vi "DataScope.vi"() -> ()   [LabVIEW 2020]
panel:
  in  "REF 종료점":u16=620
  in  "REF 시작점":u16=320
  in  "노이즈 수량":u16=255
  out "스톡스 인덱스":u32
  out "안티스톡스 인덱스":i32
  out "XY Graph":cluster{"Y":dbl[], "Y":dbl[]}[](graph) caption="XY 그래프"
  in  "거리해상도":string(combo)="5" caption="거리 해상도"
  in  "측정 거리":string(combo)="4" caption="측정 최대 거리"
  out "S문자열":string caption="스톡스 파일"
  out "AS문자열":string caption="안티스톡스 파일"
  in  "종료":bool
  in  "다음 데이터":bool
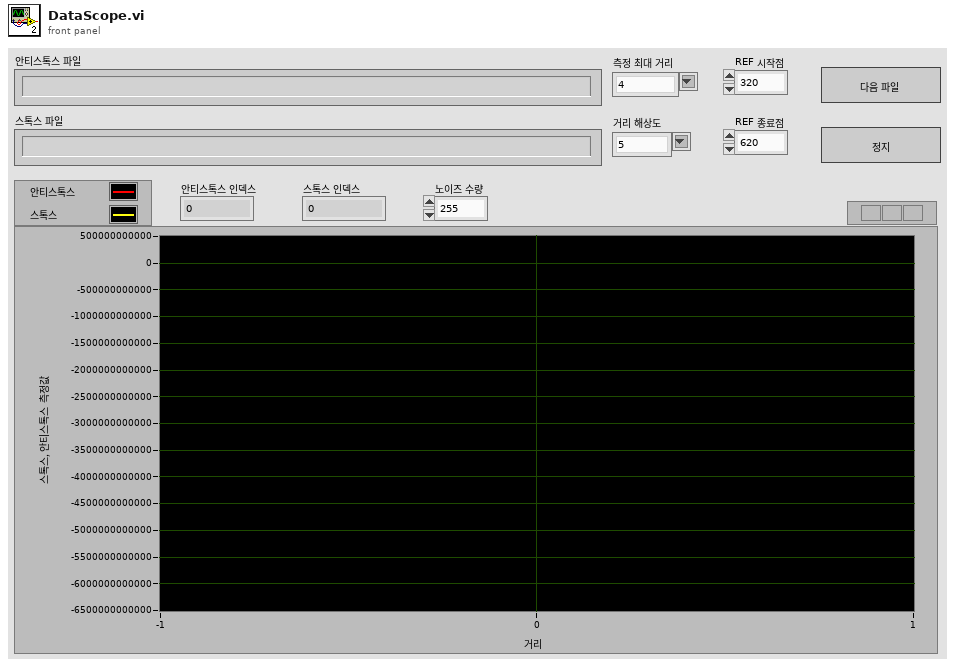
[diagram p1: front panel]
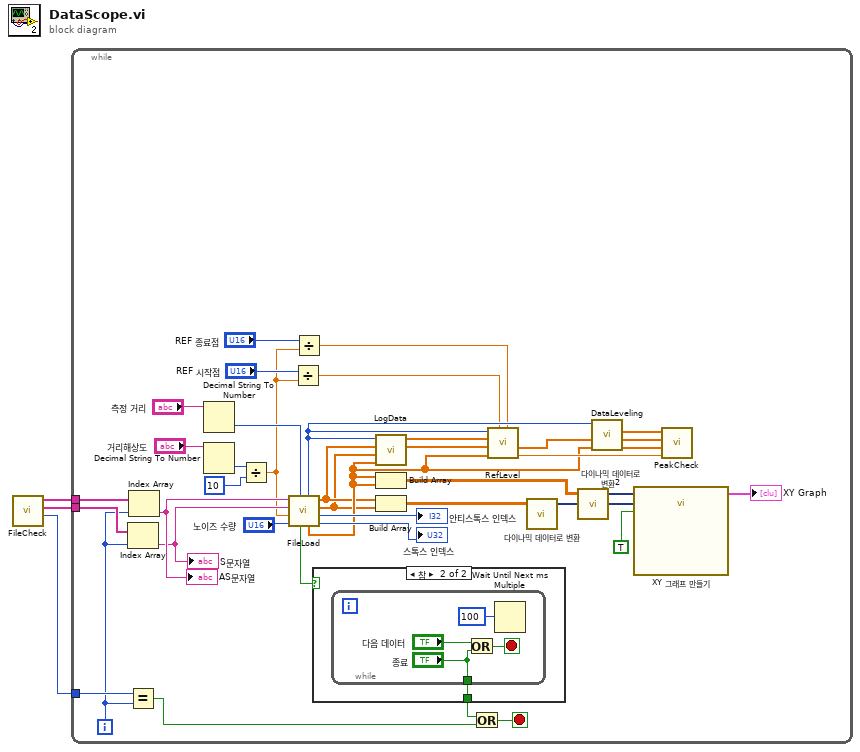
[diagram p0: block diagram]
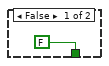
[diagram p2: hidden frame]
diagram:
  n1 = call "FileCheck.vi"() -> ("파일수"=w1:u16, "스톡스 파일 배열"=w2:string[], "안티스톡스 파일 배열"=w3:string[])  [unwired: 8 in, 1 out]
  n2 = while {
    tunnel: w3 -> [w43]
    tunnel: w2 -> [w42]
    tunnel: w1 -> [w41]
    i -> [w32]
    stop <- w28 stop-if-true
    n3 = Index Array(array=w42, index=w32) -> (element=w39:string)
    "S문자열" <- w39
    n4 = Equal?(x=w41, y=w32) -> (x = y?=w29:bool)
    n5 = Index Array(array=w43, index=w32) -> (element=w40:string)
    "AS문자열" <- w40
    n6 = Decimal String To Number(string="측정 거리") -> (number=w7:i32)  [unwired: 2 in, 1 out]
    n7 = Decimal String To Number(string="거리해상도") -> (number=w6:i32)  [unwired: 2 in, 1 out]
    n8 = Divide(x=w6, y=10) -> (x/y=w4:dbl)
    n9 = call "FileLoad.vi"("측정거리"=w7, "노이즈 수량"="노이즈 수량", "거리 해상도"=w4, "스톡스 데이터 경로 문자열"=w39, "안티스톡스 데이터 경로 문자열"=w40) -> ("스톡스 인덱스"=→"스톡스 인덱스":i32, "안티스톡스 인덱스"=→"안티스톡스 인덱스":i32, "스톡스 배열"=w16:dbl[], "안티스톡스 배열"=w17:dbl[], "거리축 배열"=w18:dbl[], "데이터 총량"=w19:u32, "대기중"=w31:bool)
    n10 = Divide(x="REF 시작점", y=w4) -> (x/y=w11:dbl)
    n11 = Divide(x="REF 종료점", y=w4) -> (x/y=w9:dbl)
    n12 = case shown="참" w31 {
      tunnel: [FALSE w45] -> w30
      frame False {
      }
      frame True {
        n13 = while {
          tunnel: ["종료"] -> w45
          stop <- w47 stop-if-true
          n14 = Or(x="다음 데이터", y="종료") -> (x .or. y?=w47:bool)
          n15 = Wait Until Next ms Multiple(millisecond multiple=100) -> ()  [unwired: 1 out]
        }
      }
    }
    n16 = call "LogData.vi"("거리 배열"=w18, "스톡스 배열"=w16, "안티스톡스 배열"=w17, "데이터 총량"=w19) -> ("LOG(S)"=w14:dbl[], "LOG(AS)"=w15:dbl[])  [unwired: 4 in, 2 out]
    n17 = Build Array(w18, w18) -> (w24:dbl[][])
    n18 = Build Array(w17, w16) -> (w34:dbl[][])
    n19 = Or(x=w30, y=w29) -> (x .or. y?=w28:bool)
    n20 = call "RefLevel.vi"("REF 종료점"=w9, "REF 시작점"=w11, "거리 배열"=w18, "Log(S) 배열"=w14, "Log(AS) 배열"=w15, "데이터 총량"=w19) -> ("REF 계산값"=w21:dbl, "Log(AS-S)"=w13:dbl[])  [unwired: 4 out]
    n21 = call "다이나믹 데이터로 변환"("2D Array"=w34) -> ("Dynamic Data Type"=w36:dynamicdata)  [unwired: 3 in]
    n22 = call "다이나믹 데이터로 변환2"("2D Array"=w24) -> ("Dynamic Data Type"=w37:dynamicdata)  [unwired: 3 in]
    n23 = call "DataLeveling.vi"("거리 배열"=w18, "LOG(AS)-LOG(S)"=w13, "데이터 총량"=w19) -> ("최종 거리 배열"=w20:dbl[], "LOG(AS)-LOG(S)"=w22:dbl[], "LOG(AS-S)"=w23:dbl[])  [unwired: 3 in, 1 out]
    n24 = call "XY 그래프 만들기"("Reset"=TRUE, "Y Input"=w36, "X Input"=w37) -> ("XY Graph"=→"XY Graph":cluster{"X":dbl[], "Y":dbl[]}[])  [unwired: 7 in, 1 out]
    n25 = call "PeakCheck.vi"("REF계산값"=w21, "거리 배열"=w20, "LOG(AS)-LOG(S)"=w22, "LOG(AS-S)"=w23) -> ()  [unwired: 7 in, 1 out]
  }
